vi "Cartesian Manipulator Inertia (Point).vi"(8 "error in (no error)":errorcluster, 10 "joint positions":dbl[](array[numeric]), 11 "serial arm in":refnum<class "NI_Robotics_Serial Robot Arm.lvclass">) -> (0 "error out":errorcluster, 2 "inertia matrix":T1, 3 "serial arm out":refnum<class "NI_Robotics_Serial Robot Arm.lvclass">)   [LabVIEW 2017, in "NI_Kinematics.lvlib"]
doc: "Calculates a matrix that represents the kinetic energy of the end effector of a robotic arm in Cartesian space. Wire data to the <B>joint positions</B> input to determine the polymorphic instance to use or manually select the instance.\n\n<B>.m file:</B> cinertia"
uses:
  <vilib>/robotics/Kinematics/NI_Kinematics.lvlib
  <vilib>/robotics/Kinematics/Robot/NI_Robotics_Serial Robot Arm.lvclass
  <vilib>/Analysis/Matrix/Datatypes/RealMatrix.ctl
  <vilib>/Analysis/7linalg.llb/Real Transpose Matrix.vi
  <vilib>/Analysis/baseanly.llb/Real A x B.vi
  <vilib>/Analysis/_algsub.llb/Real PseudoInverse Matrix.vi
  <vilib>/robotics/Kinematics/dyn/Joint Manipulator Inertia (Point).vi
  <vilib>/Analysis/NI_AALPro.lvlib
  <vilib>/Analysis/NI_AALBase.lvlib
  <vilib>/Analysis/Matrix/NI_Matrix.lvlib
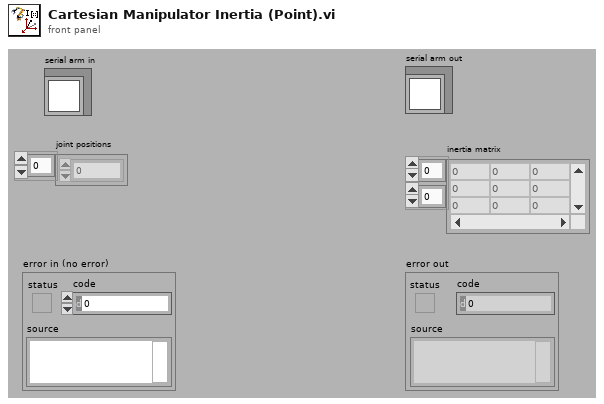
[diagram p1: front panel]
types:
  T1 = typedef "NI_Matrix.lvlib/RealMatrix.ctl" = dbl[][]
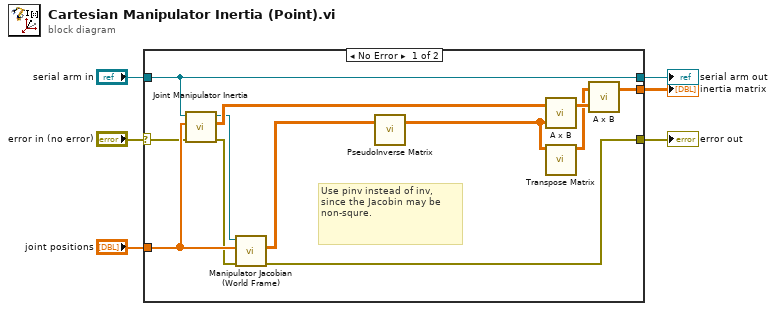
[diagram p0: block diagram]
diagram:
  n1 = case shown="No Error" "error in (no error)" {
    selector: "error in (no error)" -> [w10 w19]
    tunnel: "joint positions" -> [w18 _]
    tunnel: "serial arm in" -> [w9 w20]
    tunnel: [w14 _] -> w4
    tunnel: [w11 w19] -> w3
    tunnel: [w9 w20] -> w1
    frame No Error {
      # "Use pinv instead of inv, since the Jacobin may be non-squre."
      n2 = call-poly <vilib>:"Joint Manipulator Inertia.vi"("error in (no error)"=w10, "joint positions"=w18, "serial arm in"=w9) -> ("error out"=w12:errorcluster, "inertia matrix"=w17:T1, "serial arm out"=w13:refnum<class "NI_Robotics_Serial Robot Arm.lvclass">)  [unwired: 6 in]
      n3 = call <vilib>:"Manipulator Jacobian (World Frame).vi"("error in (no error)"=w12, "joint positions"=w18, "serial arm in"=w13) -> ("error out"=w11:errorcluster, "jacobian"=w7:T1)  [unwired: 5 in, 2 out]
      n4 = call-poly <vilib>:"PseudoInverse Matrix.vi"("Input Matrix"=w7) -> ("PseudoInverse Matrix"=w8:T1)  [unwired: 1 in, 1 out]
      n5 = call-poly <vilib>:"A x B.vi"("B"=w8, "A"=w17) -> ("A x B"=w16:T1)  [unwired: 1 out]
      n6 = call-poly <vilib>:"Transpose Matrix.vi"("Input Matrix"=w8) -> ("Matrix Transpose"=w15:T1)  [unwired: 9 in, 1 out]
      n7 = call-poly <vilib>:"A x B.vi"("B"=w16, "A"=w15) -> ("A x B"=w14:T1)  [unwired: 1 out]
    }
    frame Error {
    }
  }
  "serial arm out" <- w1
  "inertia matrix" <- w4
  "error out" <- w3
